vi "DATE WISE FOR RESON MASTER.vi"(0 "Array":string[][](array[string])=[["1999", "", "", "2", "1", "2", "2021-01-21 21:47:40", "2021-01-21 21:47:42", "2021-01-21 22:00:58", "2021-01-21 21:47:42", "2021-01-21 21:48:32", "2021-01-21 22:00:57", "224", "AAAAAAA", "", "2021-01-21", "0", "0", "", "", "", "", "", "", "", "", "", ""], ["2000", "", "", "2", "1", "2", "2021-01-21 22:07:14", "2021-01-21 22:07:15", "2021-01-21 22:08:21", "2021-01-21 22:07:15", "", "2021-01-21 22:08:20", "224", "AAAAAAA", "", "2021-01-21", "0", "0", "", "", "", "", "", "", "", "", "", ""], ["2001", "", "", "2", "1", "2", "2021-01-21 22:09:00", "2021-01-21 22:09:00", "2021-01-21 23:15:43", "2021-01-21 22:09:01", "2021-01-21 22:09:02", "2021-01-21 23:15:42", "224", "AAAAAAA", "", "2021-01-21", "0", "0", "", "", "", "", "", "", "", "", "", ""]], 3 "Select Stakeholder":string, 8 "total in date":string[](array[string])) -> (11 "COUNT OF ARRAY":dbl, 12 "Count out":string[](array[string]), 14 "DURATION":string[](array[string]), 15 "DURATION":string[](array[string]), 16 "DURATION SUM OF ARRAY":dbl, 17 "output":string[][](array[string]), 19 "error out":errorcluster)   [LabVIEW 2017]
panel:
  out "RESON ID":string[](array[string])
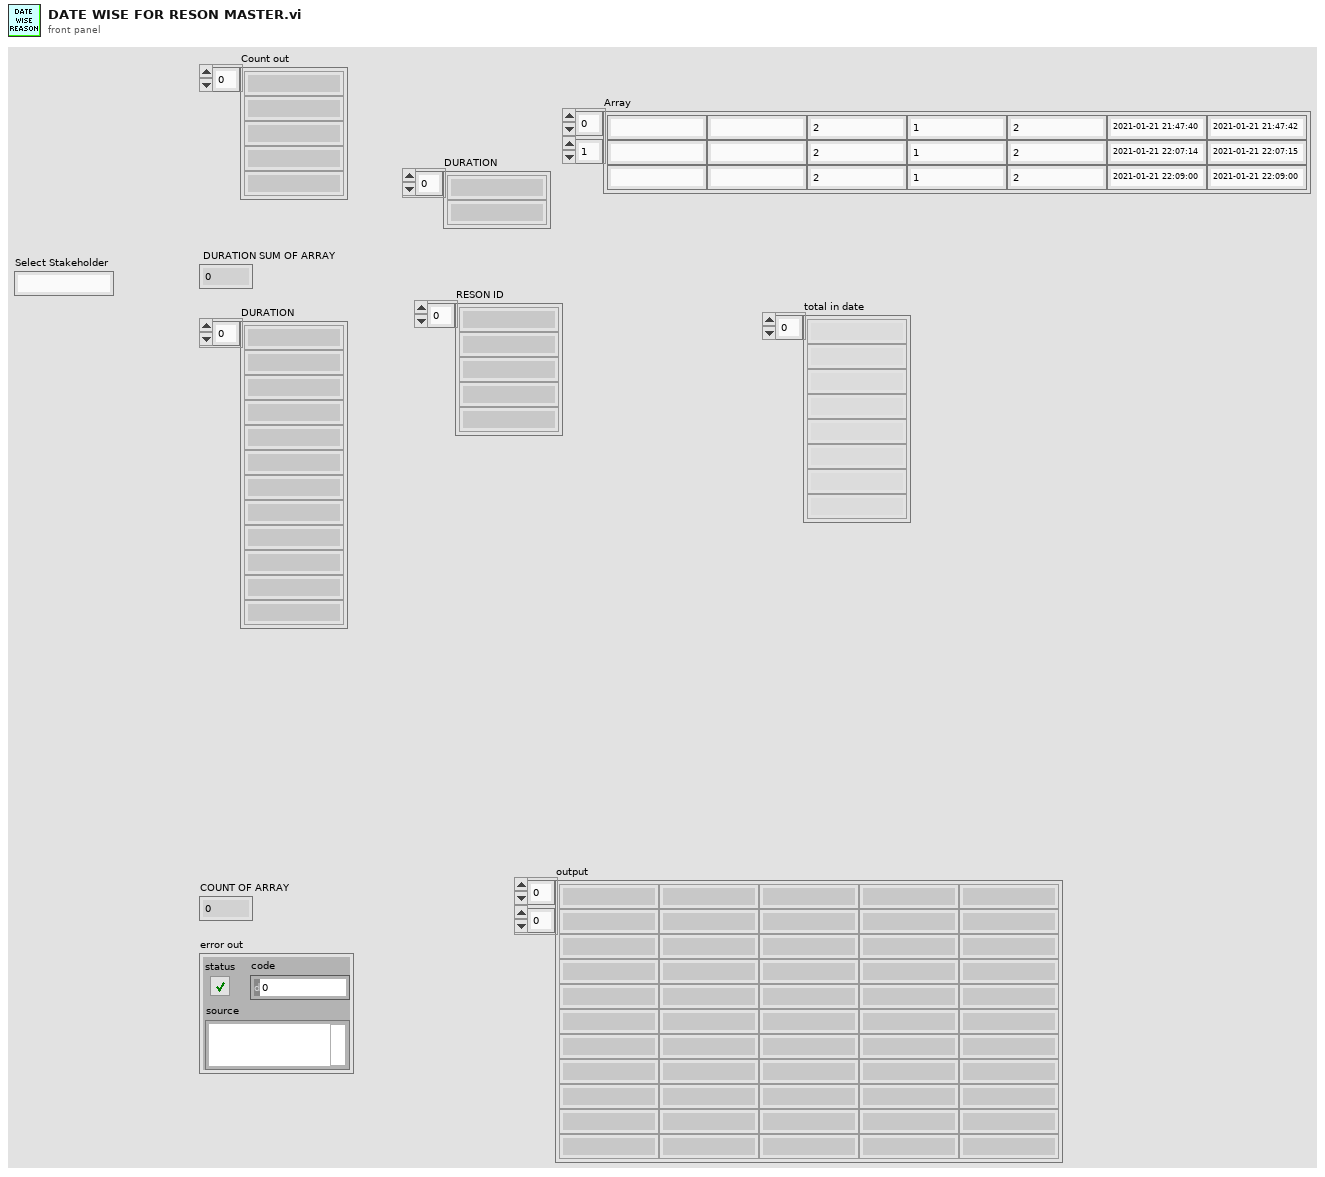
[diagram p1: front panel]
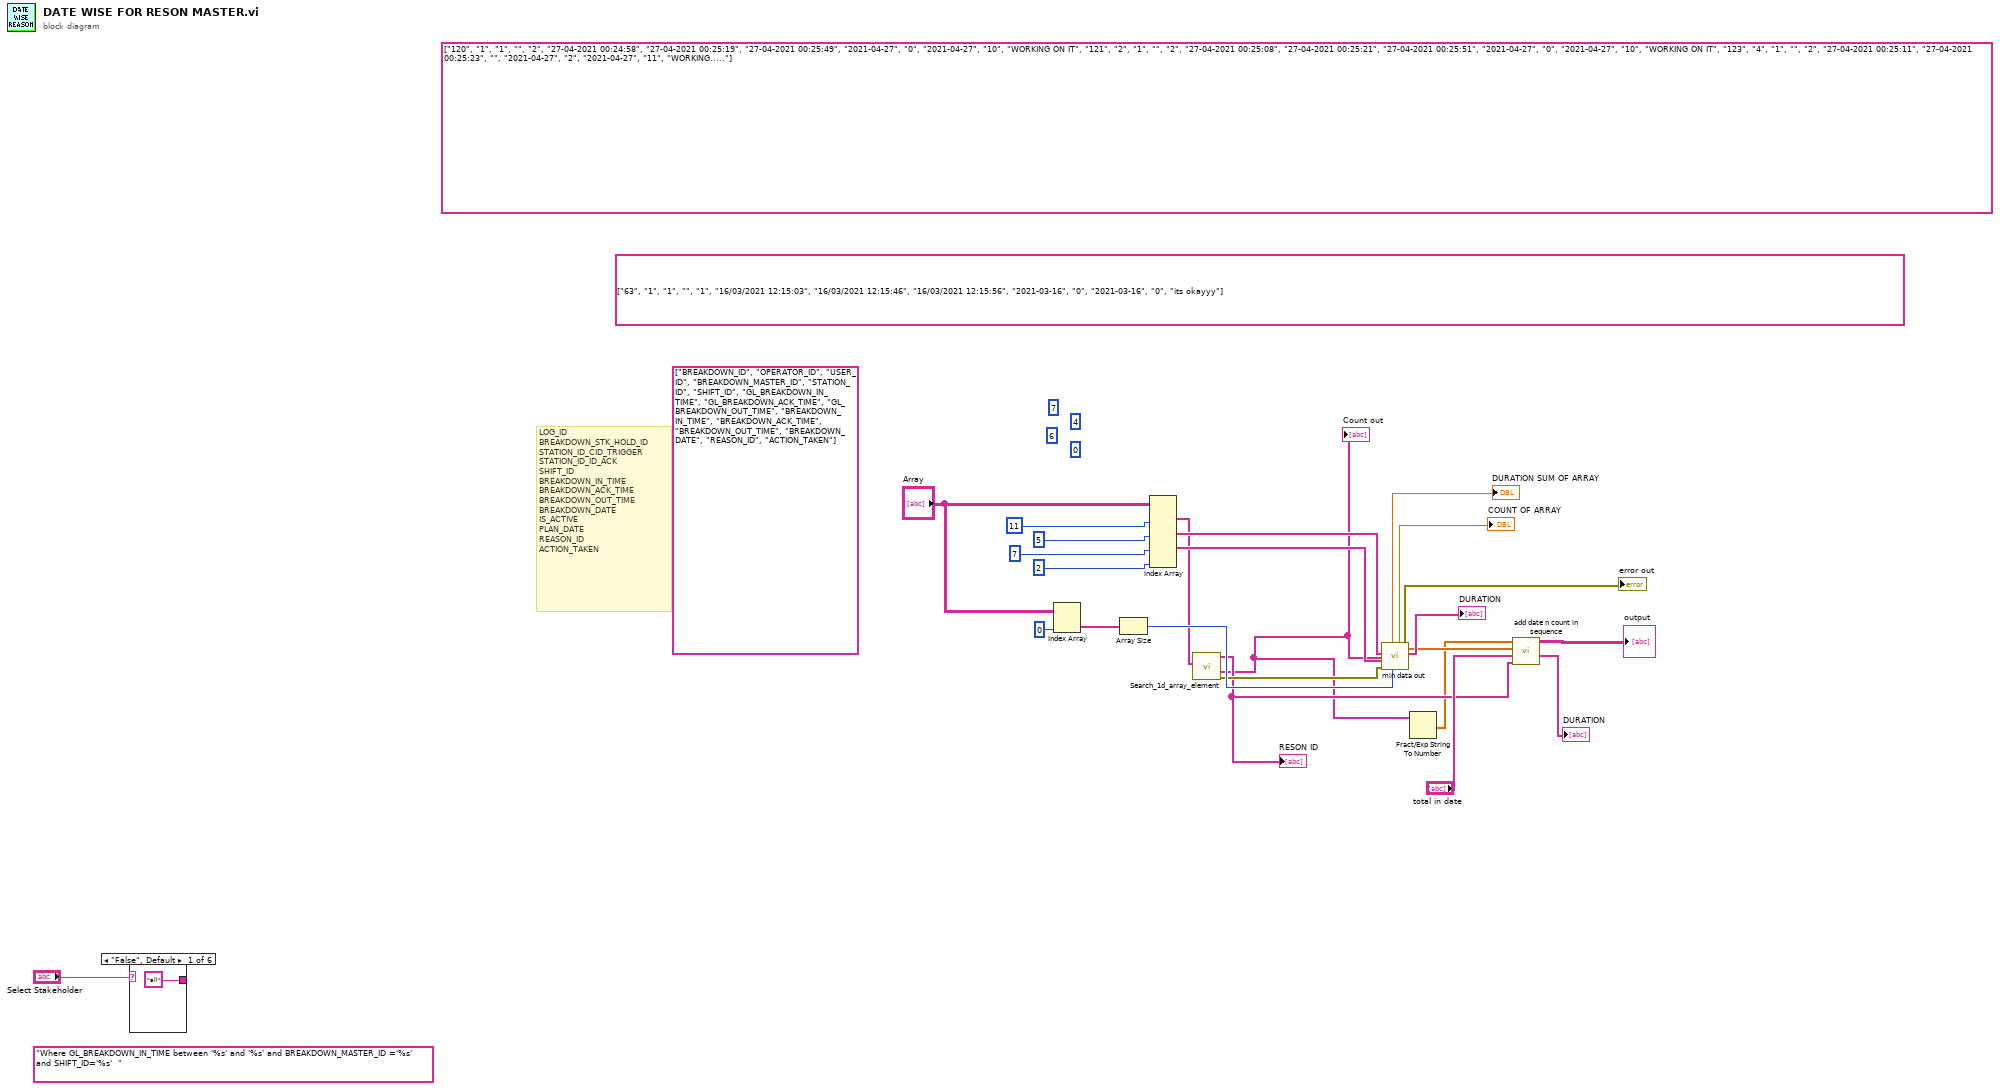
[diagram p0: block diagram]
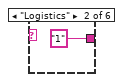
[diagram p2: hidden frame]
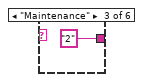
[diagram p3: hidden frame]
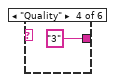
[diagram p4: hidden frame]
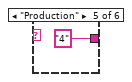
[diagram p5: hidden frame]
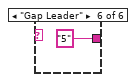
[diagram p6: hidden frame]
diagram:
  (unwired) string[][] [["120", "1", "1", "", "2", "27-04-2021 00:24:58", "27-04-2021 00:25:19", "27-04-2021 00:25:49", "2021-04-27", "0", "2021-04-27", "10", "WORKING ON IT"], ["121", "2", "1", "", "2", "27-04-2021 00:25:08", "27-04-2021 00:25:21", "27-04-2021 00:25:51", "2021-04-27", "0", "2021-04-27", "10", "WORKING ON IT"], ["123", "4", "1", "", "2", "27-04-2021 00:25:11", "27-04-2021 00:25:23", "", "2021-04-27", "2", "2021-04-27", "11", "WORKING....."]] ("Array 2")
  (unwired) string[][] [["63", "1", "1", "", "1", "16/03/2021 12:15:03", "16/03/2021 12:15:46", "16/03/2021 12:15:56", "2021-03-16", "0", "2021-03-16", "0", "its okayyy"]] ("Array")
  (unwired) string[] ["BREAKDOWN_ID", "OPERATOR_ID", "USER_ID", "BREAKDOWN_MASTER_ID", "STATION_ID", "SHIFT_ID", "GL_BREAKDOWN_IN_TIME", "GL_BREAKDOWN_ACK_TIME", "GL_BREAKDOWN_OUT_TIME", "BREAKDOWN_IN_TIME", "BREAKDOWN_ACK_TIME", "BREAKDOWN_OUT_TIME", "BREAKDOWN_DATE", "REASON_ID", "ACTION_TAKEN"] ("columns")
  (unwired) 0 ("index (col)")
  (unwired) 6 ("index (col)")
  (unwired) 4 ("index (col)")
  (unwired) 7 ("index (row)")
  (unwired) "Where GL_BREAKDOWN_IN_TIME between '%s' and '%s' and BREAKDOWN_MASTER_ID ='%s'  and SHIFT_ID='%s'  " ("condition")
  # "LOG_ID\nBREAKDOWN_STK_HOLD_ID\nSTATION_ID_CID_TRIGGER\nSTATION_ID_ID_ACK\nSHIFT_ID\nBREAKDOWN_IN_TIME\nBREAKDOWN_ACK_TIME\nBREAKDOWN_OUT_TIME\nBREAKDOWN_DATE\nIS_ACTIVE\nPLAN_DATE\nREASON_ID\nACTION_TAKEN"
  n1 = case shown="\"False\", Default" "Select Stakeholder" {
    tunnel: ["all" "1" "2" "3" "4" "5"] -> _
    frame "False", Default {
    }
    frame "Logistics" {
    }
    frame "Maintenance" {
    }
    frame "Quality" {
    }
    frame "Production" {
    }
    frame "Gap Leader" {
    }
  }
  n2 = Index Array(array="Array", index (col)=0 ("disabled index (col)")) -> (element=w18:string[])  [unwired: 1 in]
  n3 = Array Size(array=w18) -> (size(s)=w24:i32)
  n4 = Index Array(array="Array", index (col) #1=11 ("index (row)"), index (col) #2=5 ("index (col)"), index (col) #3=7 ("index (col)"), index (col) #4=2 ("index (col)")) -> (element #1=w16:string[], element #2=w19:string[], element #3=w20:string[])  [unwired: 4 in, 1 out]
  n5 = call "Search_1d_array_element.vi"("BD Date"=w16) -> ("error out"=w21:errorcluster, "Count out"=w5:string[], "Elements Found out"=w10:string[])  [unwired: 6 in]
  "RESON ID" <- w10
  "Count out" <- w5
  n6 = call "min data out.vi"("Numeric"=w24, "error in (no error)"=w21, "out time"=w20, "in time"=w19, "Count in"=w5) -> ("error out"=→"error out":errorcluster, "string min"=→"DURATION":string[], "duration"=w11:dbl[], "COUNT OF ARRAY"=→"COUNT OF ARRAY":dbl, "DURATION SUM OF ARRAY"=→"DURATION SUM OF ARRAY":dbl)  [unwired: 2 in]
  n7 = Fract/Exp String To Number(string=w5) -> (number=w9:dbl[])  [unwired: 3 in, 1 out]
  n8 = call "add date n count in sequence.vi"("find date"=w10, "total date"="total in date", "duration"=w11, "count"=w9) -> ("DURATION"=→"DURATION":string[], "appended array"=→"output":string[][])  [unwired: 5 in, 1 out]
